vi "Read Characters From File with Error Out.vi"(0 "file path (dialog if empty)":path, 1 "convert eol? (no:F)":bool, 5 "number of characters (all:-1)":i32=-1, 7 "start of read offset (chars.:0)":i32, 9 "start path (Not A Path)":path=path "", 13 "[pattern]":string) -> (4 "new file path (NotAPath if cancelled)":path, 6 "character string":string, 8 "mark after read (chars.)":i32, 10 "EOF?":bool, 15 "error out":errorcluster)   [LabVIEW 2019]
doc: "Reads a specified number of characters from a byte stream file beginning at a specified character offset."
panel:
  in  "prompt":string="Choose file to read."
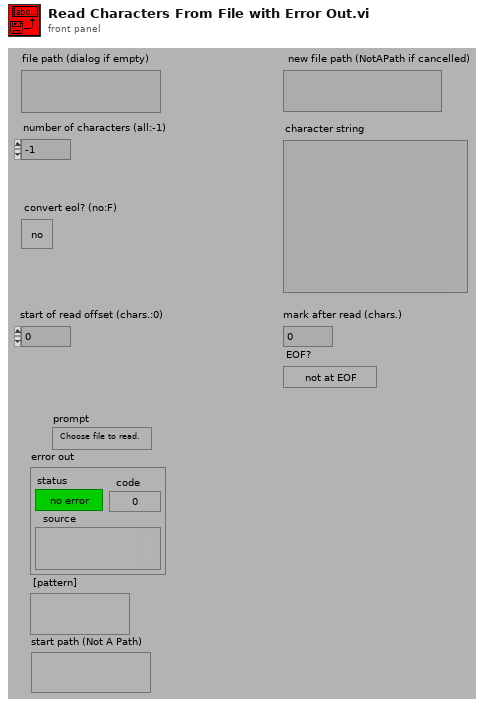
[diagram p1: front panel]
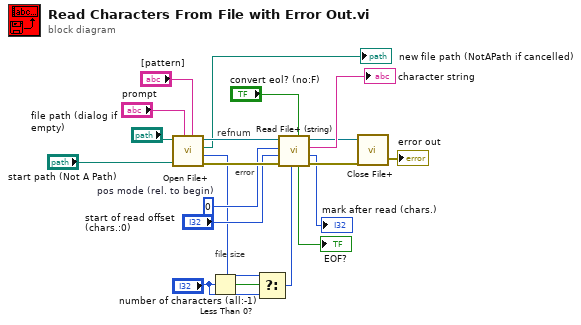
[diagram p0: block diagram]
diagram:
  w17 = i16 0  # pos mode (rel. to begin)
  # "file size"
  # "error"
  # "refnum"
  n1 = call <vilib>:"Open File+.vi"("[pattern]"="[pattern]", "prompt"="prompt", "start path (Not A Path)"="start path (Not A Path)", "file path (\" \")"="file path (dialog if empty)") -> ("error out"=w19:errorcluster, "file size (bytes)"=w8:i32, "file path"=→"new file path (NotAPath if cancelled)":path, "refnum"=w11:refnum<file>)  [unwired: 4 in]
  n2 = Less Than 0?(x="number of characters (all:-1)") -> (x < 0?=w9:bool)
  n3 = Select(t=w8, s=w9, f="number of characters (all:-1)") -> (s? t:f=w6:i32)
  n4 = call <vilib>:"Read File+ (string).vi"("convert eol? (no:F)"="convert eol? (no:F)", "count"=w6, "error in (no error)"=w19, "pos offset (bytes:0)"="start of read offset (chars.:0)", "pos mode (rel. to current:2)"=w17, "refnum"=w11) -> ("error out"=w15:errorcluster, "mark after read (bytes)"=→"mark after read (chars.)":i32, "string"=→"character string":string, "dup refnum"=w14:refnum<file>, "EOF?"=→"EOF?":bool)  [unwired: 1 in]
  n5 = call <vilib>:"Close File+.vi"("error in (no error)"=w15, "refnum"=w14) -> ("error out"=→"error out":errorcluster)  [unwired: 3 in, 2 out]
